vi "Scan Timestamp.vi"(8 "error in (no error)":errorcluster, 11 "String":string) -> (0 "error out":errorcluster, 3 "Timestamp":timestamp)   [LabVIEW 2020, in "Library Commun.lvlib" / "JSON Scalar.lvclass"]
uses:
  JSON Scalar.lvclass
  JSON Scalar.lvclass/JSON Scalar.ctl
panel:
  out "remaining string":string
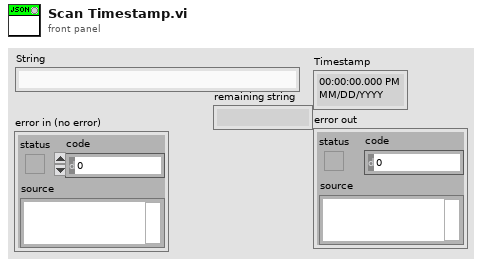
[diagram p1: front panel]
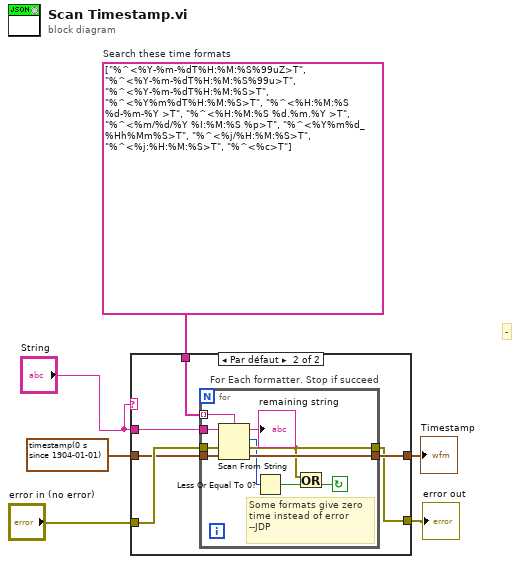
[diagram p0: block diagram]
diagram:
  w6 = string[] ["%^<%Y-%m-%dT%H:%M:%S%99uZ>T", "%^<%Y-%m-%dT%H:%M:%S%99u>T", "%^<%Y-%m-%dT%H:%M:%S>T", "%^<%Y%m%dT%H:%M:%S>T", "%^<%H:%M:%S %d-%m-%Y >T", "%^<%H:%M:%S %d.%m.%Y >T", "%^<%m/%d/%Y %I:%M:%S %p>T", "%^<%Y%m%d_%Hh%Mm%S>T", "%^<%j/%H:%M:%S>T", "%^<%j:%H:%M:%S>T", "%^<%c>T"]  # Search these time formats
  # "-"
  n1 = case shown="Par défaut" "String" {
    tunnel: [w7 w14] -> w1
    tunnel: "error in (no error)" -> [w8 w13]
    tunnel: [w8 w12] -> w3
    tunnel: timestamp(0 s since 1904-01-01) ("default value 1") -> [w7 w11]
    tunnel: "String" -> [_ w10]
    tunnel: w6 -> [_ w9]
    frame "null" {
    }
    frame Default {
      n2 = for "For Each formatter. Stop if succeed" {
        tunnel: [w24] -> w14
        tunnel: w13 -> [w23]
        tunnel: [w17] -> w12
        tunnel: w11 -> [w22]
        tunnel: w10 -> [w21]
        tunnel: w9 -> [w20] mode=indexing
        stop <- w18 continue-if-true
        # "Some formats give zero\ntime instead of error\n--JDP"
        n3 = Scan From String(format string=w20, input string=w21, error in=w23, default 1=w22) -> (remaining string=→"remaining string":string, offset past scan=w16:u32, error out=w17:errorcluster, output 1=w24:timestamp)  [unwired: 1 in]
        n4 = Less Or Equal To 0?(x=w16) -> (x <= 0?=w19:bool)
        n5 = Or(x=w17, y=w19) -> (x .or. y?=w18:bool)
      }
    }
  }
  "error out" <- w3
  "Timestamp" <- w1
